vi "midi-tracks.get_number.vi"(8 "error in (no error)":errorcluster, 11 "midi-file-events in":refnum<class "midi-file-events.lvclass">) -> (0 "error out":errorcluster, 2 "Numer of Tracks":i32, 3 "midi-file-events out":refnum<class "midi-file-events.lvclass">)   [LabVIEW 2020, in "midi-file-events.lvclass"]
uses:
  midi-file-events.lvclass
  midi-file-events.lvclass/midi-file-events.ctl
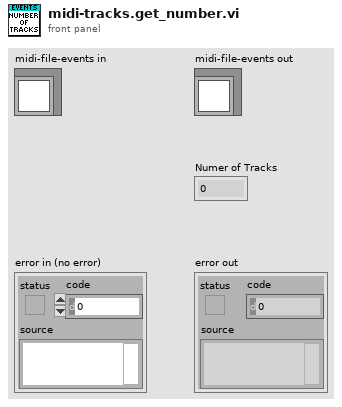
[diagram p1: front panel]
types:
  T1 = map{i32, refnum<class "midi-file-event.lvclass">[]}
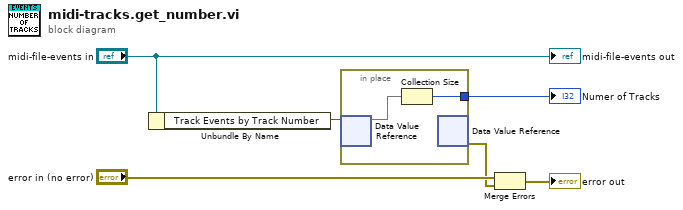
[diagram p0: block diagram]
diagram:
  n1 = Unbundle By Name("midi-file-events in") -> ("Track Events by Track Number"=w6:refnum<data-value>)
  n2 = in-place {
    in-place-border: [w7] -> w5
    n3 = in-place-dvr #1(w6) -> (w8:T1)  [unwired: 1 out]
    n4 = Collection Size(1:w8) -> (0:w7:i32)
    n5 = in-place-dvr #1() -> (w2:errorcluster)  [unwired: 1 in, 1 out]
  }
  "Numer of Tracks" <- w5
  n6 = Merge Errors("error in (no error)", w2) -> (→"error out":errorcluster)
  "midi-file-events out" <- "midi-file-events in"
